vi "Generate AnalogOutput.vi"(8 "error in (no error)":errorcluster, 10 "Output Value":dbl, 11 "Rack Pin":string) -> (0 "error out":errorcluster)   [LabVIEW 2024, in "Shared Steps.lvlib"]
uses:
  Shared Steps.lvlib
  <vilib>/DAQmx/write.llb/DAQmx Write (Analog DBL 1Chan 1Samp).vi
  <vilib>/DAQmx/create/channels.llb/DAQmx Create Channel (AO-Voltage-Basic).vi
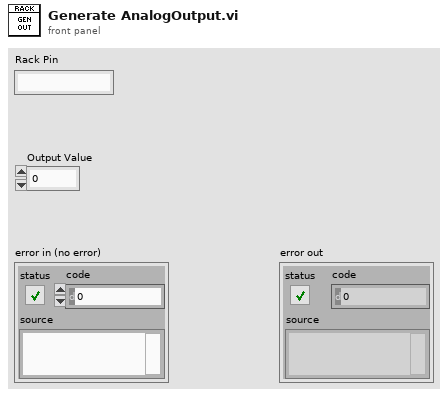
[diagram p1: front panel]
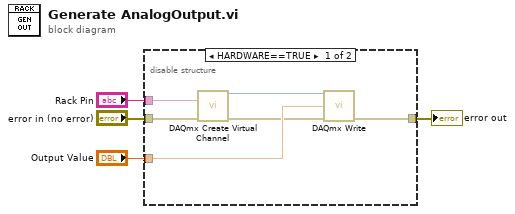
[diagram p0: block diagram]
diagram:
  n1 = disable-structure shown="HARDWARE==TRUE" {
    disable-tunnel: "Rack Pin" -> [w10 _]
    disable-tunnel: "Output Value" -> [w9 _]
    disable-tunnel: "error in (no error)" -> [w6 w11]
    disable-tunnel: [w5 w11] -> w1
    frame condition #0 {
      n2 = call-poly <vilib>:"DAQmx Create Virtual Channel.vi"("physical channels"=w10, "error in"=w6) -> ("task out"=w8:refnum<k21>, "error out"=w7:errorcluster)  [unwired: 12 in]
      n3 = call-poly <vilib>:"DAQmx Write.vi"("task/channels in"=w8, "data"=w9, "error in"=w7) -> ("error out"=w5:errorcluster)  [unwired: 10 in, 2 out]
    }
    frame condition #1 (active) {
    }
  }
  "error out" <- w1
